vi "Wasapi_out_in.vi"(6 "error play 4":errorcluster, 7 "信号时长":dbl caption="等待时间（秒）" format="%#_6p", 8 "Format":cluster{"Rate":i32, "Bits":i32, "Channels":u32}={"Rate"=44100, "Bits"=32, "Channels"=2}, 9 "card #":u32, 10 "data_length":i32, 11 "output data":i32[][](array[numeric])) -> (2 "error play 2":errorcluster, 3 "error play 3":errorcluster, 4 "MIC_Data_IN":dbl[][](array[numeric]))   [LabVIEW 2018]
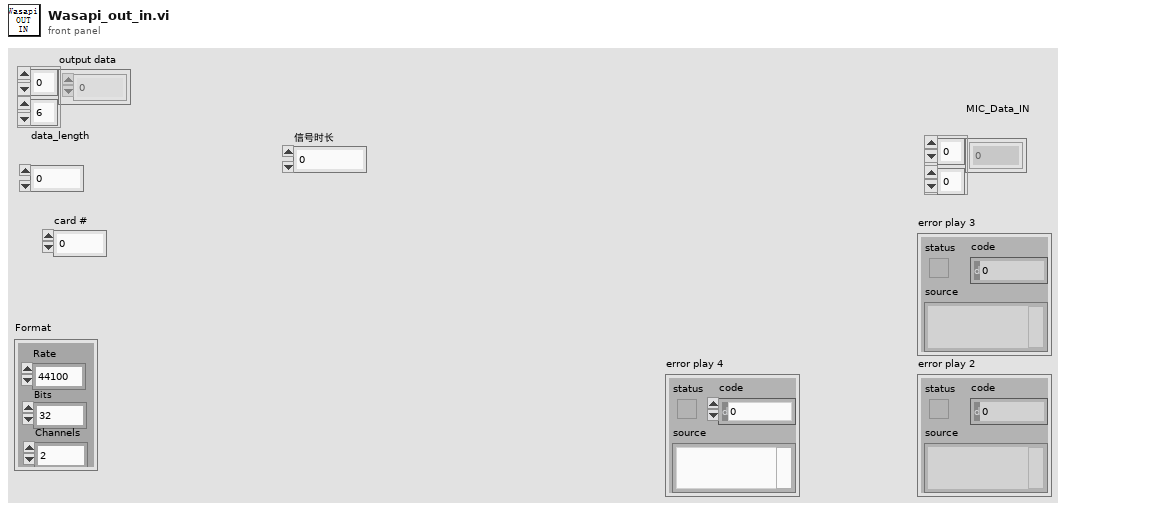
[diagram p1: front panel]
types:
  T1 = cluster{"# buffers":i32, "Buffer size":i32, "unit (ms)":enum16{"time (ms)", "Samples"}}
  T2 = typedef "SoundHandle.ctl" = cluster{"DeviceID":u16, "Samples/buf":u32, "Sampl rate":u32, "Bits/sample":u16, "Channels":u8, "Opened":bool}
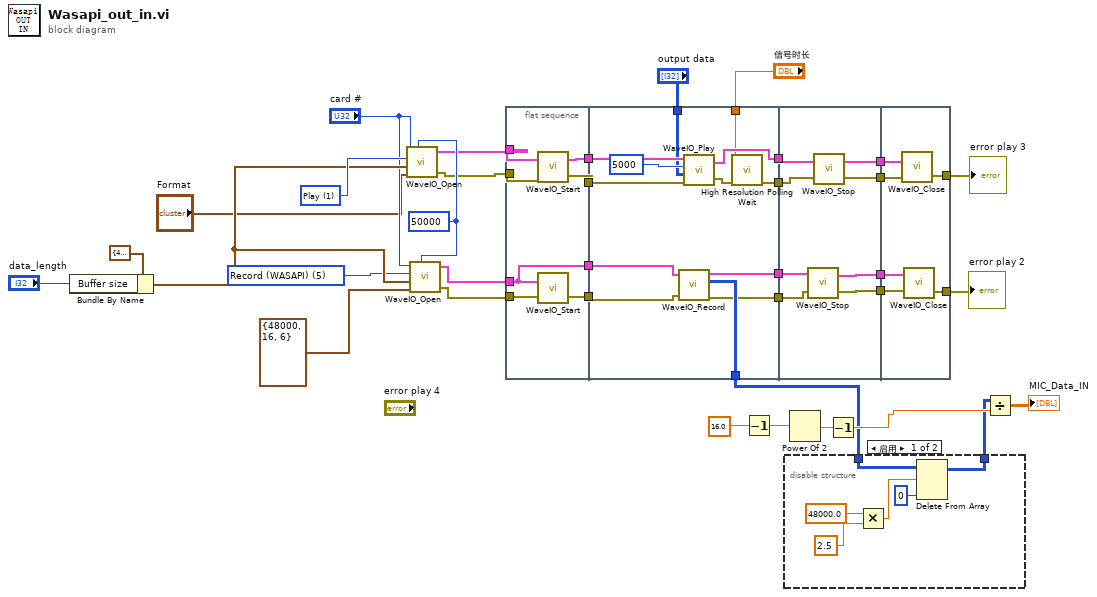
[diagram p0: block diagram]
diagram:
  w24 = u16 1 items=["Record", "Play", "Loopback", "ASIO input", "ASIO output", "Record (WASAPI)", "Play (WASAPI)", "Record Combi", "Play Combi"] ("device type (Record)")
  w18 = u16 5 items=["Record", "Play", "Loopback", "ASIO input", "ASIO output", "Record (WASAPI)", "Play (WASAPI)", "Record Combi", "Play Combi"] ("device type (Record)")
  w21 = 50000 ("Watchdog timeout (msec) (default=OFF)")
  n1 = Bundle By Name(cluster=T1 {"# buffers"=4, "Buffer size"=88200, "unit (ms)"=enum."Samples"} ("Buffer"), "Buffer size"="data_length") -> (w23:T1)
  n2 = call "WaveIO_Open.vi"("idev"="card #", "Watchdog timeout (msec) (default=OFF)"=w21, "device type (Record)"=w24, "Buffer Config"=w23, "Format (44kHz, 16Bit, stereo)"="Format") -> ("Sound Handle Out"=w15:T2, "error out"=w16:errorcluster)  [unwired: 2 in]
  n3 = call "WaveIO_Open.vi"("idev"="card #", "Watchdog timeout (msec) (default=OFF)"=w21, "device type (Record)"=w18, "Buffer Config"=w23, "Format (44kHz, 16Bit, stereo)"=cluster{"Rate":i32, "Bits":i32, "Channels":u32} {"Rate"=48000, "Bits"=16, "Channels"=6}) -> ("Sound Handle Out"=w17:T2, "error out"=w8:errorcluster)  [unwired: 2 in]
  n4 = flat-sequence {
    tunnel: [w40] -> w36
    tunnel: [w41] -> w35
    tunnel: w16 -> [w43]
    tunnel: w15 -> [w42]
    tunnel: w8 -> [w39]
    tunnel: w17 -> [w38]
    tunnel: [w38] -> w34
    tunnel: [w37] -> w33
    tunnel: [w51] -> w32
    tunnel: [w52] -> w31
    tunnel: w36 -> [w56]
    tunnel: w35 -> [w55]
    tunnel: w34 -> [w50]
    tunnel: w33 -> [w44]
    tunnel: [w49] -> w6
    tunnel: [w48] -> w30
    tunnel: [w47] -> w29
    tunnel: "信号时长" -> [w46]
    tunnel: "output data" -> [w45]
    tunnel: w32 -> [w60]
    tunnel: w31 -> [w59]
    tunnel: w30 -> [w64]
    tunnel: w29 -> [w63]
    tunnel: [w62] -> w28
    tunnel: [w61] -> w27
    tunnel: [w58] -> w26
    tunnel: [w57] -> w25
    tunnel: w28 -> [w70]
    tunnel: w27 -> [w69]
    tunnel: [w68] -> w14
    tunnel: w26 -> [w67]
    tunnel: w25 -> [w66]
    tunnel: [w65] -> w20
    frame #0 {
      n5 = call "WaveIO_Start.vi"("error in (no error)"=w43, "Handle"=w42) -> ("error out"=w41:errorcluster, "Handle Out"=w40:T2)
      n6 = call "WaveIO_Start.vi"("error in (no error)"=w39, "Handle"=w38) -> ("error out"=w37:errorcluster)  [unwired: 1 out]
    }
    frame #1 {
      n7 = call "WaveIO_Record.vi"("Handle"=w50, "error in (no error)"=w44) -> ("Handle Out"=w48:T2, "Data"=w49:i32[][], "error out"=w47:errorcluster)  [unwired: 1 in, 2 out]
      n8 = call "WaveIO_Play.vi"("error in (no error)"=w55, "data"=w45, "timeout (automatic)"=5000, "Handle"=w56) -> ("error out"=w53:errorcluster, "Handle Out"=w51:T2)
      n9 = call <vilib>:"High Resolution Polling Wait.vi"("error in (no error)"=w53, "seconds to wait"=w46) -> ("error out"=w52:errorcluster)  [unwired: 9 in]
    }
    frame #2 {
      n10 = call "WaveIO_Stop.vi"("error in (no error)"=w63, "Handle"=w64) -> ("error out"=w61:errorcluster, "Handle Out"=w62:T2)
      n11 = call "WaveIO_Stop.vi"("error in (no error)"=w59, "Handle"=w60) -> ("error out"=w57:errorcluster, "Handle Out"=w58:T2)
    }
    frame #3 {
      n12 = call "WaveIO_Close.vi"("error in (no error)"=w66, "Handle"=w67) -> ("error out"=w65:errorcluster)  [unwired: 1 out]
      n13 = call "WaveIO_Close.vi"("error in (no error)"=w69, "Handle"=w70) -> ("error out"=w68:errorcluster)  [unwired: 1 out]
    }
  }
  n14 = Decrement(x=16.0) -> (x-1=w1:dbl)
  n15 = disable-structure shown="启用" {
    disable-tunnel: w6 -> [w73 w77]
    disable-tunnel: [w71 w77] -> w5
    frame Enabled {
      n16 = Multiply(x=48000.0, y=2.5) -> (x*y=w72:dbl)
      n17 = Delete From Array(array=w73, length=w72, index (col)=0 ("禁用的索引 (列)")) -> (array with subset deleted=w71:i32[][])  [unwired: 1 in, 1 out]
    }
    frame Disabled {
    }
  }
  n18 = Power Of 2(x=w1) -> (2^x=w13:dbl)
  n19 = Decrement(x=w13) -> (x-1=w12:dbl)
  n20 = Divide(x=w5, y=w12) -> (x/y=→"MIC_Data_IN":dbl[][])
  "error play 2" <- w14
  "error play 3" <- w20
